vi "Set port.vi"(8 "error in (no error)":errorcluster, 9 "Value":string, 10 "Puerto":dbl, 11 "Simulado in":refnum<class "Simulado.lvclass">) -> (0 "error out":errorcluster, 3 "Simulado out":refnum<class "Simulado.lvclass">)   [LabVIEW 2020, in "Simulado.lvclass"]
uses:
  Simulado.lvclass
  Simulado.lvclass/Simulado.ctl
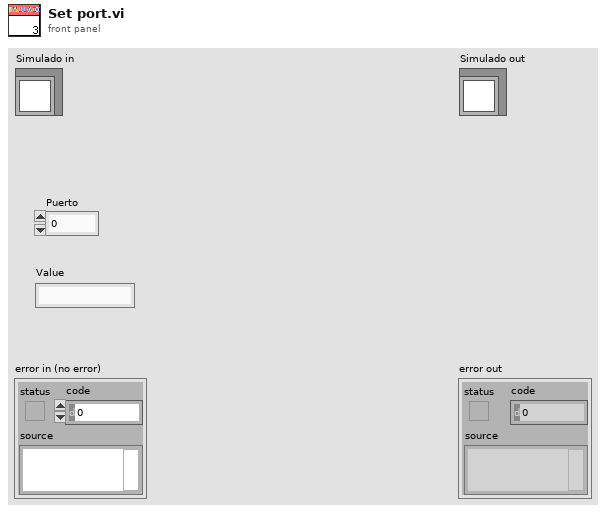
[diagram p1: front panel]
types:
  T1 = enum16{"reset parameters", "Get parameters", "Set parameter"}
  T2 = typedef "Serial Device.lvclass/serial device brand.ctl" = string
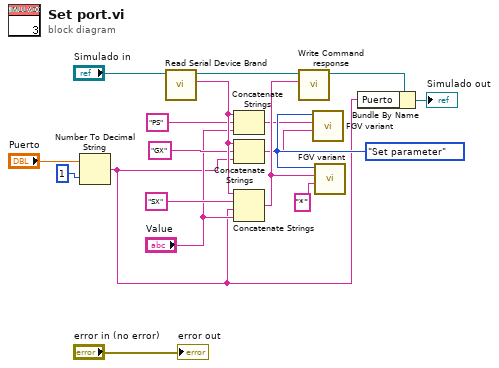
[diagram p0: block diagram]
diagram:
  w10 = T1."Set parameter" ("Functions")
  n1 = Number To Decimal String(number="Puerto", width (-)=i16 1) -> (decimal integer string=w1:string)
  n2 = call-dynamic "Read Serial Device Brand.vi"("Serial Device in"="Simulado in") -> ("Serial Device Brand"=w5:T2, "Serial Device out"=w15:refnum<class "Simulado.lvclass">)  [unwired: 8 in, 1 out]
  n3 = Concatenate Strings(w5, "PS" ("string"), "Value") -> (w6:string)
  n4 = Concatenate Strings(w5, "GX" ("string"), w1) -> (w7:string)
  n5 = Concatenate Strings(w5, "SX" ("string"), w1, "Value") -> (w9:string)
  n6 = call-dynamic "Write Command response.vi"("Command response"=w9, "Simulado in"=w15) -> ("Simulado out"=w14:refnum<class "Simulado.lvclass">)  [unwired: 8 in, 1 out]
  n7 = call "FGV variant.vi"("Response to save"=w7, "Command"=w6, "Functions"=w10) -> ()  [unwired: 7 in, 2 out]
  n8 = call "FGV variant.vi"("Response to save"="*", "Command"=w9, "Functions"=w10) -> ()  [unwired: 7 in, 2 out]
  n9 = Bundle By Name(cluster=w14, "Puerto"=w1) -> (→"Simulado out":refnum<class "Simulado.lvclass">)
  "error out" <- "error in (no error)"
